vi "GetFixtureSerialNumber.vi"(0 "name or relative path":string="ModisEdgeScanner.ini", 3 "error in (no error)":errorcluster) -> (7 "Fixture Serial Number":string, 8 "OK":bool, 10 "error out":errorcluster)   [LabVIEW 2015]
uses:
  <vilib>/Utility/config.llb/Read Key (String).vi
  <vilib>/Utility/config.llb/Write Key (String).vi
  <vilib>/Utility/config.llb/NI_LVConfig.lvlib
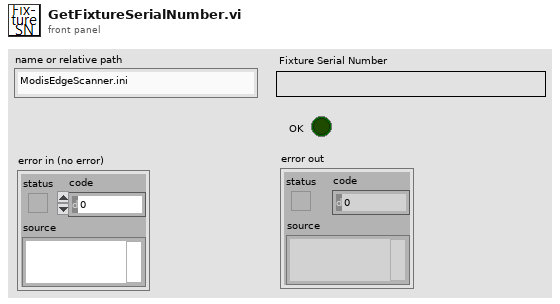
[diagram p1: front panel]
types:
  T1 = typedef "NI_LVConfig.lvlib/Config Data RefNum.ctl" = refnum<k1>
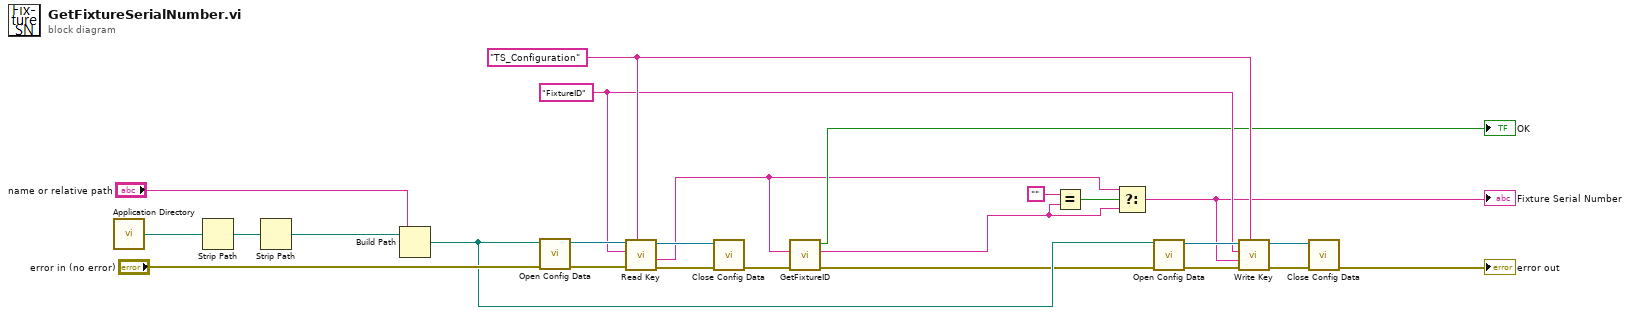
[diagram p0: block diagram]
diagram:
  w16 = "TS_Configuration" ("section")
  w15 = "FixtureID" ("key")
  n1 = call <vilib>:"Application Directory.vi"() -> ("Application Directory"=w10:path)
  n2 = Strip Path(path=w10) -> (stripped path=w2:path)  [unwired: 1 out]
  n3 = Strip Path(path=w2) -> (stripped path=w1:path)  [unwired: 1 out]
  n4 = Build Path(base path=w1, name or relative path="name or relative path") -> (appended path=w12:path)
  n5 = call <vilib>:"Open Config Data.vi"("error in (no error)"="error in (no error)", "configuration file path"=w12) -> ("error out"=w21:errorcluster, "refnum"=w24:T1)  [unwired: 7 in, 1 out]
  n6 = call-poly <vilib>:"Read Key.vi"("section"=w16, "error in (no error)"=w21, "key"=w15, "refnum"=w24) -> ("error out"=w22:errorcluster, "value"=w3:string, "refnum out"=w23:T1)  [unwired: 4 in, 1 out]
  n7 = call <vilib>:"Close Config Data.vi"("error in (no error)"=w22, "refnum"=w23) -> ("error out"=w9:errorcluster)  [unwired: 8 in, 1 out]
  n8 = call "GetFixtureID.vi"("error in (no error)"=w9, "Current Fixture ID :"=w3) -> ("error out"=w8:errorcluster, "Fixture Serial Number"=w4:string, "OK"=→"OK":bool)  [unwired: 7 in]
  n9 = Equal?(x="", y=w4) -> (x = y?=w6:bool)
  n10 = Select(t=w3, s=w6, f=w4) -> (s? t:f=w5:string)
  "Fixture Serial Number" <- w5
  n11 = call <vilib>:"Open Config Data.vi"("error in (no error)"=w8, "configuration file path"=w12) -> ("error out"=w19:errorcluster, "refnum"=w18:T1)  [unwired: 7 in, 1 out]
  n12 = call-poly <vilib>:"Write Key.vi"("section"=w16, "error in (no error)"=w19, "value"=w5, "key"=w15, "refnum"=w18) -> ("error out"=w20:errorcluster, "refnum out"=w17:T1)  [unwired: 4 in, 1 out]
  n13 = call <vilib>:"Close Config Data.vi"("error in (no error)"=w20, "refnum"=w17) -> ("error out"=→"error out":errorcluster)  [unwired: 8 in, 1 out]
